vi "SubVI_Verificar_angulo_3_encontrado.vi"(1 "menor que, dê certo (graus)":dbl, 2 "maior que, dê certo (graus)":dbl, 3 "Angulo encontrado em Rad":dbl) -> (0 "Resultado(Rad)":dbl)   [LabVIEW 2017]
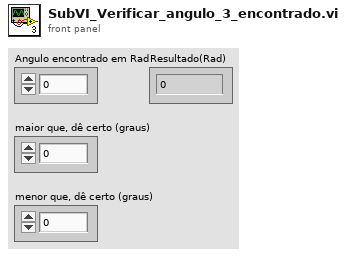
[diagram p1: front panel]
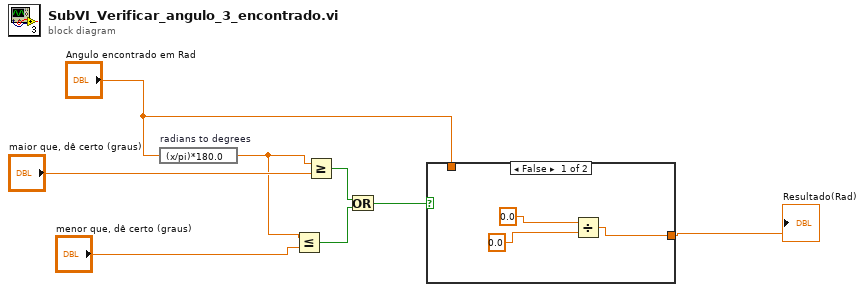
[diagram p0: block diagram]
diagram:
  n1 = expression code="(x/pi)*180.0" "radians to degrees"("Angulo encontrado em Rad") -> (w4:dbl)
  n2 = Less Or Equal?(x=w4, y="menor que, dê certo (graus)") -> (x <= y?=w2:bool)
  n3 = Greater Or Equal?(x=w4, y="maior que, dê certo (graus)") -> (x >= y?=w1:bool)
  n4 = Or(x=w1, y=w2) -> (x .or. y?=w6:bool)
  n5 = case shown="False" w6 {
    tunnel: [w9 w12] -> w7
    tunnel: "Angulo encontrado em Rad" -> [_ w12]
    frame False {
      n6 = Divide(x=0.0, y=0.0) -> (x/y=w9:dbl)
    }
    frame True {
    }
  }
  "Resultado(Rad)" <- w7
